vi "personirijillas.vi"() -> ()   [LabVIEW 2013]
uses:
  <vilib>/silver_ctls/ArrayMatrixCluster/Real Matrix NI_Silver.ctl
  <vilib>/Platform/portaccess.llb/Out Port8.vi
  <vilib>/Platform/portaccess.llb/In Port8.vi
  <vilib>/Platform/portaccess.llb/Out Port32.vi
panel:
  in  "stop":bool
  out "-14":bool
  out "16":bool
  out "-17":bool
  out "-1":bool
  out "10":bool
  out "-11":bool
  out "12":bool
  out "13":bool
  out "15":bool
  out "2 2":bool
  out "3 2":bool
  out "4 2":bool
  out "5 2":bool
  out "6":bool
  out "7":bool
  out "8":bool
  out "9":bool
  in  "Puerto":i16(ring)=888 items=["3BC"=956, "378"=888, "278"=632]
  in  "Actualizar cada (ms)":u32=100
  in  "CONTROL":i8 format="%08b"
  out "STATUS":i8 format="%08b"
  out "Real Matrix 2":T1
  out "Command":string
  out "5":bool
  out "4":bool
  out "3":bool
  out "2":bool
  out "1":bool
  out "Reconocida":dbl[](graph)
  out "Input Signal Energy":dbl
  out "Entrada":waveform(dbl)[](graph)
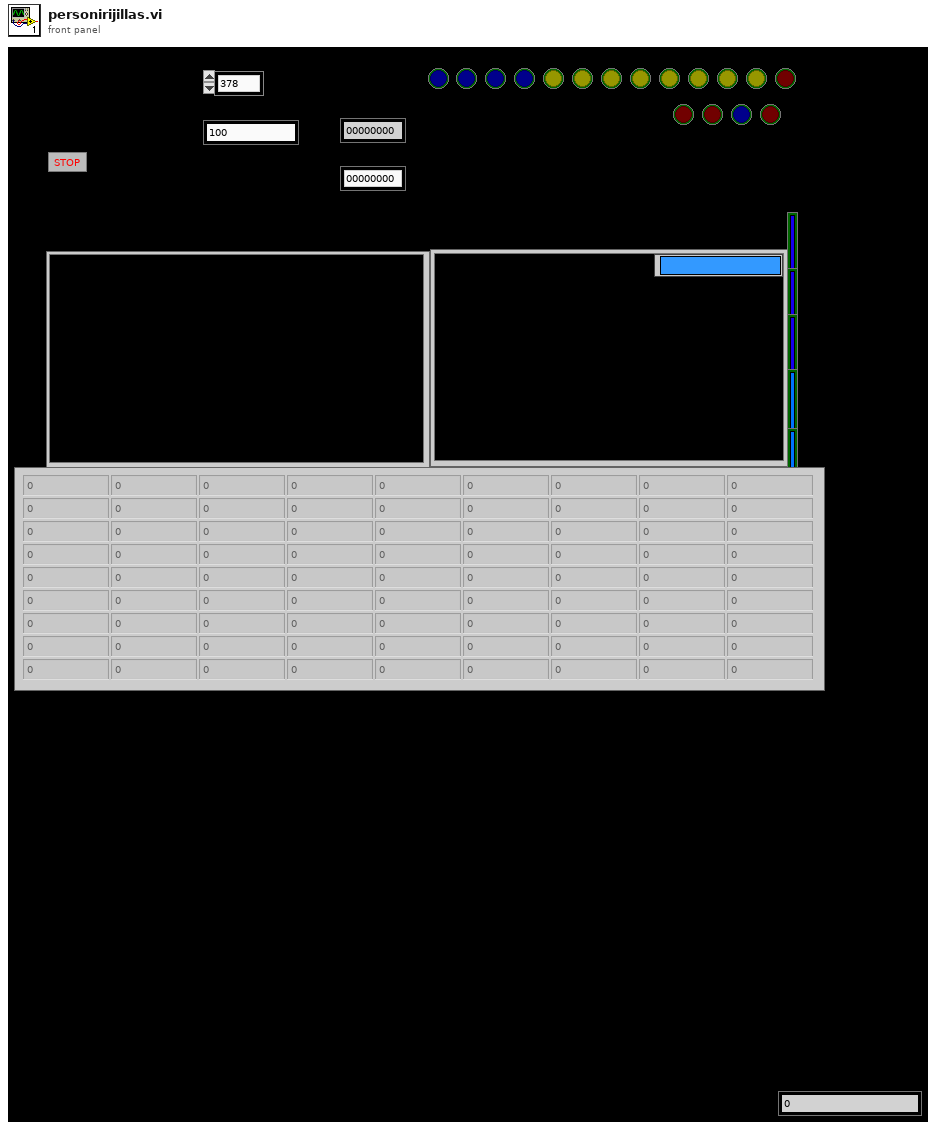
[diagram p1: front panel]
types:
  T1 = typedef "Real Matrix NI_Silver.ctl" = dbl[][]
  T2 = cluster{"Boolean array[0]":bool, "Boolean array[1]":bool, "Boolean array[2]":bool, "Boolean array[3]":bool, "Boolean array[4]":bool, "Boolean array[5]":bool, "Boolean array[6]":bool, "Boolean array[7]":bool, "Boolean array[8]":bool}
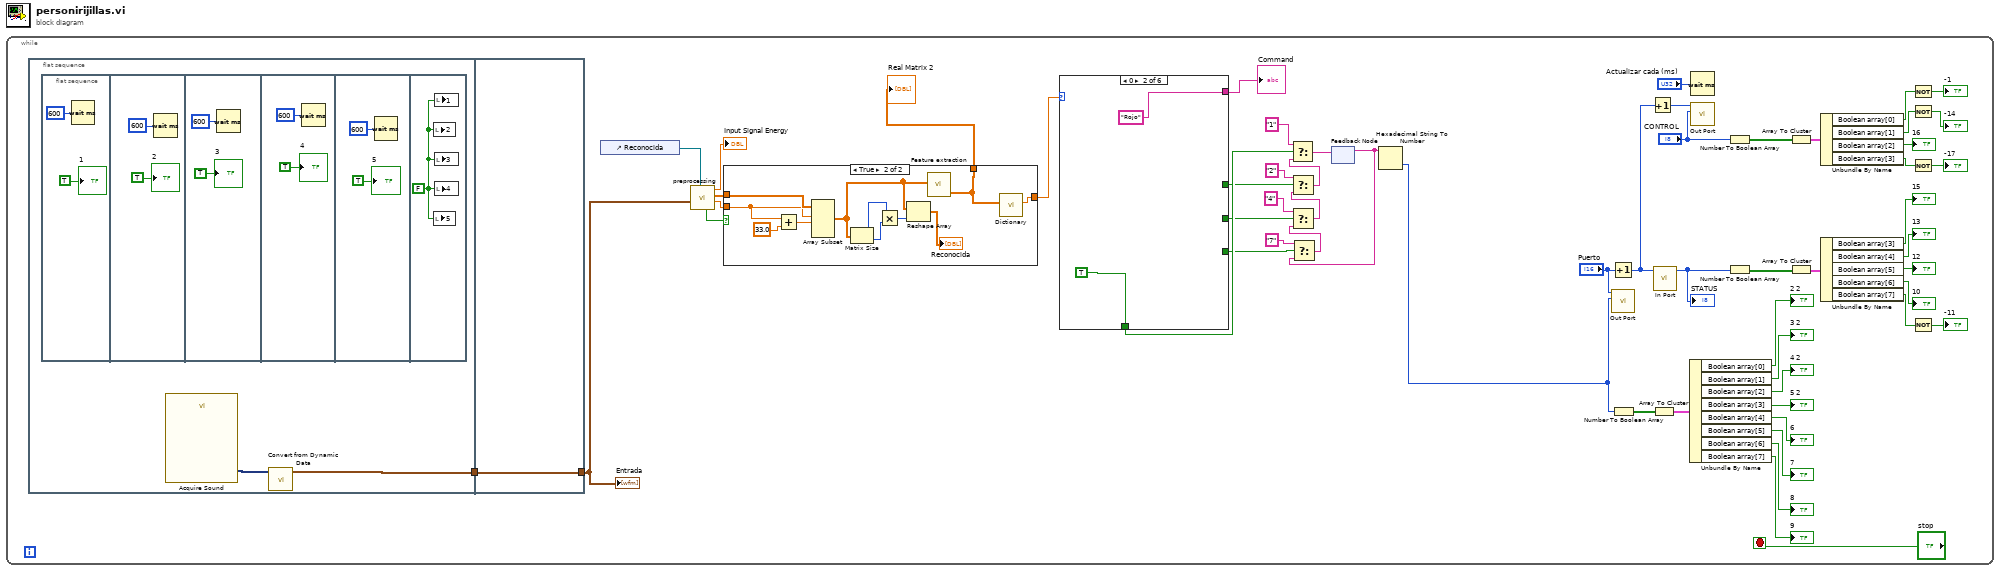
[diagram p0: block diagram]
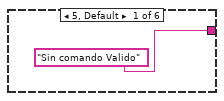
[diagram p2: hidden frame]
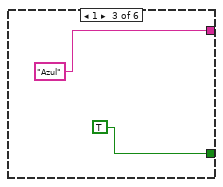
[diagram p3: hidden frame]
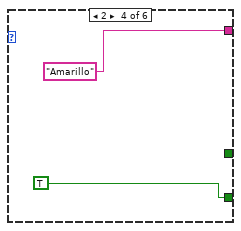
[diagram p4: hidden frame]
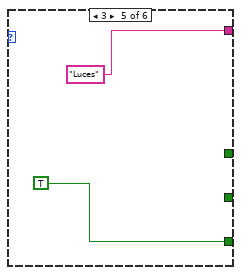
[diagram p5: hidden frame]
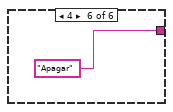
[diagram p6: hidden frame]
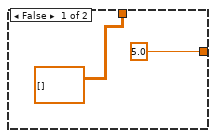
[diagram p7: hidden frame]
diagram:
  n1 = while {
    stop <- "stop" stop-if-true
    n2 = flat-sequence {
      tunnel: [w82] -> w54
      tunnel: [w95] -> w52
      tunnel: w54 -> [w95]
      frame #0 {
        n3 = flat-sequence {
          frame #0 {
            n4 = Wait (ms)(milliseconds to wait=u32 600) -> ()  [unwired: 1 out]
            "1" <- TRUE ("1")
          }
          frame #1 {
            n5 = Wait (ms)(milliseconds to wait=u32 600) -> ()  [unwired: 1 out]
            "2" <- TRUE ("1")
          }
          frame #2 {
            n6 = Wait (ms)(milliseconds to wait=u32 600) -> ()  [unwired: 1 out]
            "3" <- TRUE ("1")
          }
          frame #3 {
            n7 = Wait (ms)(milliseconds to wait=u32 600) -> ()  [unwired: 1 out]
            "4" <- TRUE ("1")
          }
          frame #4 {
            n8 = Wait (ms)(milliseconds to wait=u32 600) -> ()  [unwired: 1 out]
            "5" <- TRUE ("1")
          }
          frame #5 {
            w94 = FALSE ("1")
            n9 = local write "2"(w94) -> ()
            n10 = local write "5"(w94) -> ()
            n11 = local write "1"(w94) -> ()
            n12 = local write "3"(w94) -> ()
            n13 = local write "4"(w94) -> ()
          }
        }
        n14 = call "Acquire Sound"() -> ("Data"=w83:dynamicdata)  [unwired: 18 in, 1 out]
        n15 = call "Convert from Dynamic Data"("Dynamic Data Type"=w83) -> ("Array of Waveform"=w82:waveform(dbl)[])  [unwired: 3 in]
      }
      frame #1 {
      }
    }
    n16 = control-ref of="Reconocida"() -> (w51:refnum<vi>)
    n17 = call "preprocessing.vi"("WaveformGraph in"=w51, "Input Speech"=w52) -> ("Start index"=w57:dbl, "Frames"=w56:dbl[][], "Signal energy"=→"Input Signal Energy":dbl, "Boolean"=w58:bool)  [unwired: 6 in]
    n18 = case shown="True" w58 {
      tunnel: w57 -> [_ w74]
      tunnel: w56 -> [_ w75]
      tunnel: [5.0 ("Best Match") w73] -> w55
      tunnel: [dbl[][] [] ("Acoustic vector") w71] -> w50
      frame False {
      }
      frame True {
        n19 = Add(x=w74, y=33.0 ("x")) -> (x+y=w80:dbl)
        n20 = Array Subset(array=w75, index (row)=w74, length (row)=w80) -> (w72:dbl[][])  [unwired: 2 in]
        n21 = Matrix Size(0:w72) -> (1:w79:i32, 2:w78:i32)
        n22 = Multiply(x=w79, y=w78) -> (x*y=w77:i32)
        n23 = Reshape Array(w72, w77) -> (→"Reconocida":dbl[])
        n24 = call "Feature extraction.vi"("Utterance Frames"=w72) -> ("Acoustic vector"=w71:dbl[][])  [unwired: 10 in]
        n25 = call "Dictionary.vi"("Match Input"=w71) -> ("Best Match"=w73:dbl)  [unwired: 10 in]
      }
    }
    "Real Matrix 2" <- w50
    n26 = case shown="0" w55 {
      tunnel: [_ TRUE ("RIGHT") _ _ _ _] -> w13
      tunnel: ["Sin comando Valido" ("Command") "Rojo" ("Command") "Azul" ("Command") "Amarillo" ("Command") "Luces" ("Command") "Apagar" ("Command")] -> w49
      tunnel: [_ _ TRUE ("RIGHT") _ _ _] -> w8
      tunnel: [_ _ _ TRUE ("RIGHT") _ _] -> w7
      tunnel: [_ _ _ _ TRUE ("RIGHT") _] -> w4
      frame 5, Default {
      }
      frame 0 {
      }
      frame 1 {
      }
      frame 2 {
      }
      frame 3 {
      }
      frame 4 {
      }
    }
    "Command" <- w49
    n27 = feedback #1() -> (w1:string)  [unwired: 1 in]
    n28 = Select(t="7" ("Command"), s=w4, f=w1) -> (s? t:f=w6:string)
    n29 = Select(t="4" ("Command"), s=w7, f=w6) -> (s? t:f=w10:string)
    n30 = Select(t="2" ("Command"), s=w8, f=w10) -> (s? t:f=w12:string)
    n31 = Select(t="1" ("Command"), s=w13, f=w12) -> (s? t:f=w2:string)
    n32 = feedback-in #1(w2) -> ()
    n33 = Hexadecimal String To Number(string=w1) -> (number=w3:u32)  [unwired: 2 in, 1 out]
    n34 = Increment(x="Puerto") -> (x+1=w43:i16)
    n35 = call-poly <vilib>:"Out Port.vi"("write value"=w3, "address"="Puerto") -> ()  [unwired: 1 in, 7 out]
    n36 = Number To Boolean Array(number=w3) -> (Boolean array=w42:bool[])
    n37 = Increment(x=w43) -> (x+1=w47:i16)
    n38 = Array To Cluster(array=w42) -> (cluster=w41:T2)
    n39 = call-poly <vilib>:"In Port.vi"("address"=w43) -> ("data read"=w45:i8)  [unwired: 1 in, 7 out]
    "STATUS" <- w45
    n40 = Unbundle By Name(w41) -> ("Boolean array[0]"=→"2 2":bool, "Boolean array[1]"=→"3 2":bool, "Boolean array[2]"=→"4 2":bool, "Boolean array[3]"=→"5 2":bool, "Boolean array[4]"=→"6":bool, "Boolean array[5]"=→"7":bool, "Boolean array[6]"=→"8":bool, "Boolean array[7]"=→"9":bool)
    n41 = Wait (ms)(milliseconds to wait="Actualizar cada (ms)") -> ()  [unwired: 1 out]
    n42 = call-poly <vilib>:"Out Port.vi"("write value"="CONTROL", "address"=w47) -> ()  [unwired: 1 in, 7 out]
    n43 = Number To Boolean Array(number="CONTROL") -> (Boolean array=w37:bool[])
    n44 = Number To Boolean Array(number=w45) -> (Boolean array=w39:bool[])
    n45 = Array To Cluster(array=w37) -> (cluster=w38:T2)
    n46 = Array To Cluster(array=w39) -> (cluster=w40:T2)
    n47 = Unbundle By Name(w38) -> ("Boolean array[0]"=w17:bool, "Boolean array[1]"=w19:bool, "Boolean array[2]"=→"16":bool, "Boolean array[3]"=w21:bool)
    n48 = Unbundle By Name(w40) -> ("Boolean array[3]"=→"15":bool, "Boolean array[4]"=→"13":bool, "Boolean array[5]"=→"12":bool, "Boolean array[6]"=→"10":bool, "Boolean array[7]"=w23:bool)
    n49 = Not(x=w17) -> (.not. x?=→"-1":bool)
    n50 = Not(x=w19) -> (.not. x?=→"-14":bool)
    n51 = Not(x=w21) -> (.not. x?=→"-17":bool)
    n52 = Not(x=w23) -> (.not. x?=→"-11":bool)
    "Entrada" <- w52
  }
